vi "Test.vi"() -> ()   [LabVIEW 2017]
doc: "This example shows how to create, run a script and query the script output data."
uses:
  <instrlib>/Keithley 2600 Series/Keithley 2600 Series.lvlib
panel:
  out "Graph 2":cluster{"Y":dbl[], "Y":dbl[]}[](graph)
  out "Current":string
  in  "Numeric":i32=6000
  out "Voltage":string
  out "Time":string
  in  "Source Code":string="smua.reset()\nsmua.source.limitv = 1\nSweepILinMeasureV(smua, 0.01, 0.1, 0.2, 10)\nprintbuffer(1, 10, smua.nvbuffer1)\nprint(smua.nvbuffer1.readings[10])\n"
  in  "Script Variable (myScript)":string="myScript"
  in  "VISA resource name":refnum<visa-resource-name>
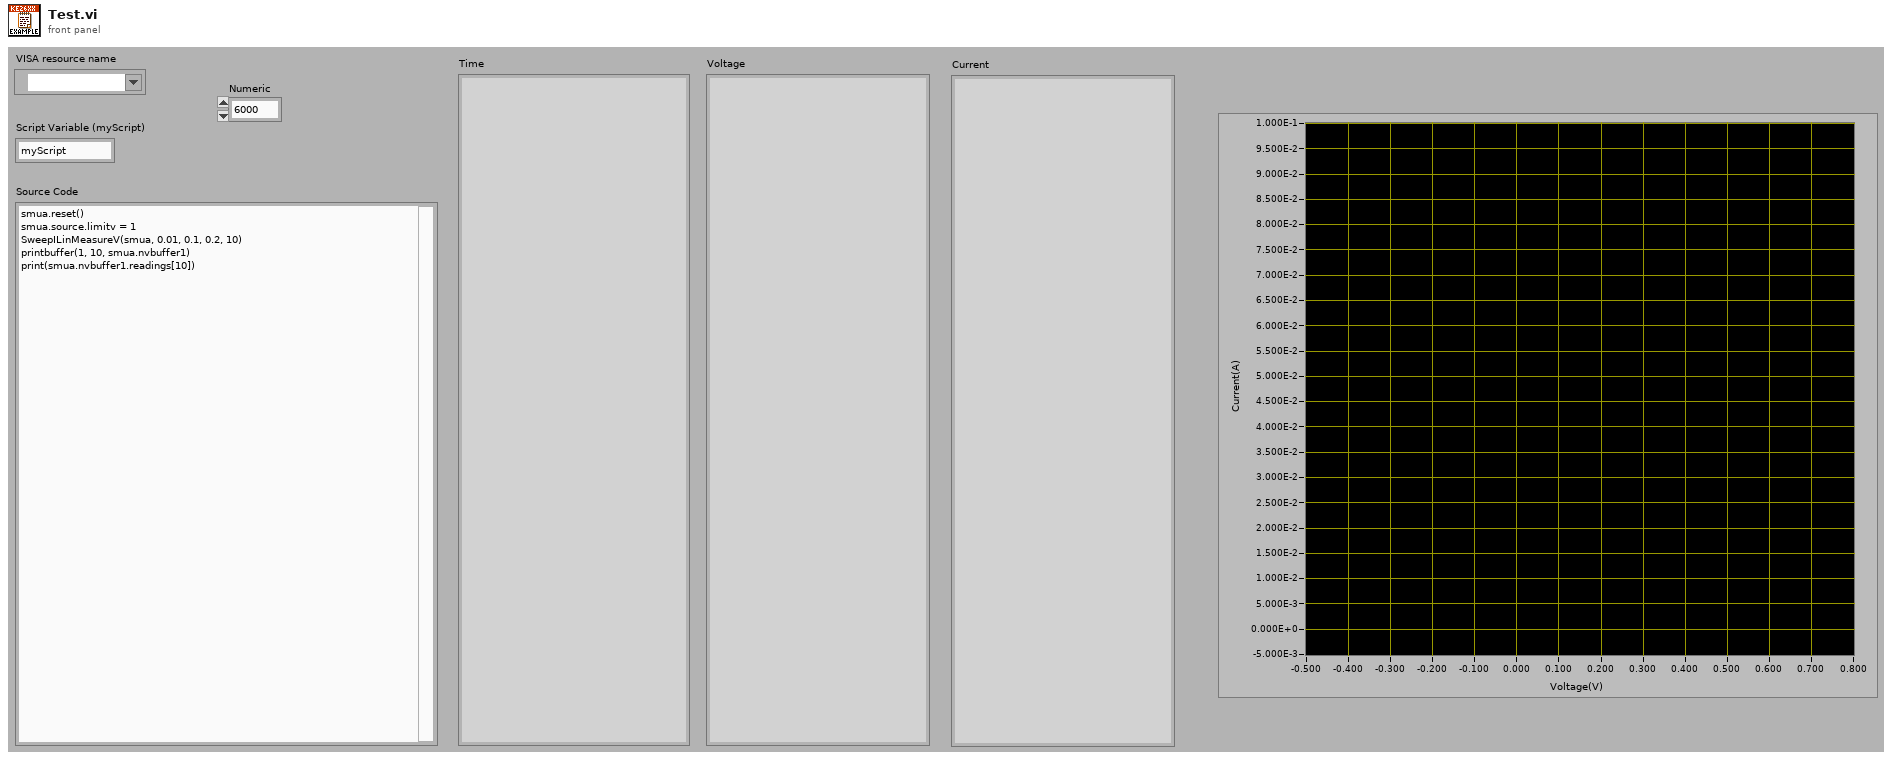
[diagram p1: front panel]
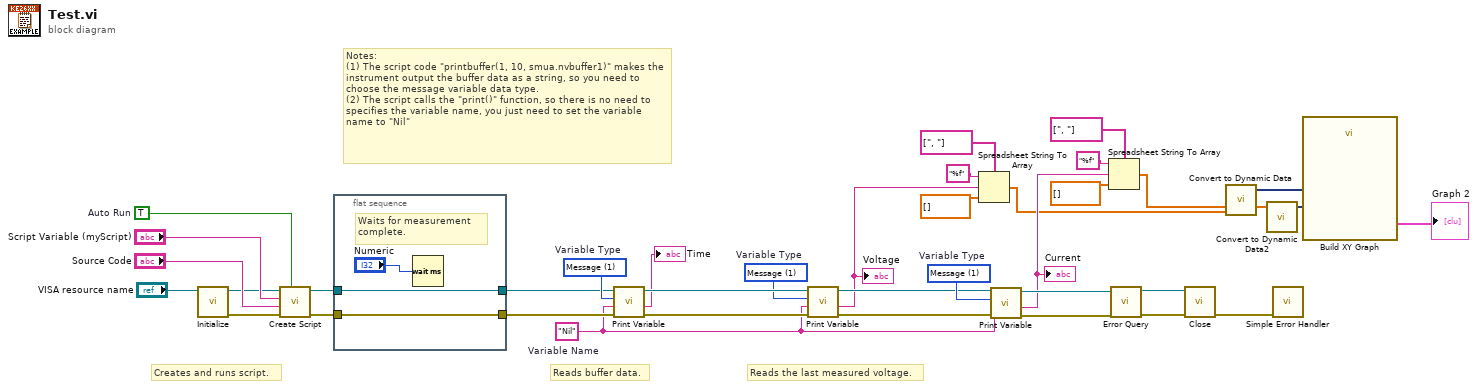
[diagram p0: block diagram]
diagram:
  w19 = 1 items=["Number", "Message"]  # Variable Type
  w30 = 1 items=["Number", "Message"]  # Variable Type
  w33 = 1 items=["Number", "Message"]  # Variable Type
  w14 = "Nil"  # Variable Name
  w34 = TRUE  # Auto Run
  # "Reads buffer data."
  # "Reads the last measured voltage."
  # "Notes: \n(1) The script code \"printbuffer(1, 10, smua.nvbuffer1)\" makes the instrument output the buffer data as a string, so you need to choose the message variable data type.\n(2) The script calls the \"print()\" function, so there is no need to specifies the variable name, you just need to set the variable name to \"Nil\""
  # "Creates and runs script."
  n1 = call <instrlib>:"Initialize.vi"("VISA resource name"="VISA resource name") -> ("error out"=w20:errorcluster, "VISA resource name out"=w21:refnum<visa-resource-name>)  [unwired: 9 in]
  n2 = call <instrlib>:"Create Script.vi"("Auto Run (F: Disable)"=w34, "error in (no error)"=w20, "Source Code"="Source Code", "Script Variable"="Script Variable (myScript)", "VISA resource name"=w21) -> ("error out"=w28:errorcluster, "VISA resource name out"=w29:refnum<visa-resource-name>)  [unwired: 5 in]
  n3 = flat-sequence {
    tunnel: w29 -> [w38]
    tunnel: w28 -> [w39]
    tunnel: [w39] -> w26
    tunnel: [w38] -> w27
    frame #0 {
      # "Waits for measurement complete."
      n4 = Wait (ms)(milliseconds to wait="Numeric") -> ()  [unwired: 1 out]
    }
  }
  n5 = call <instrlib>:"Print Variable.vi"("error in (no error)"=w26, "Variable Name"=w14, "Variable Type (0: Number)"=w33, "VISA resource name"=w27) -> ("error out"=w31:errorcluster, "Message"=→"Time":string, "VISA resource name out"=w32:refnum<visa-resource-name>)  [unwired: 4 in, 1 out]
  n6 = call <instrlib>:"Print Variable.vi"("error in (no error)"=w31, "Variable Name"=w14, "Variable Type (0: Number)"=w30, "VISA resource name"=w32) -> ("error out"=w16:errorcluster, "Message"=w11:string, "VISA resource name out"=w18:refnum<visa-resource-name>)  [unwired: 4 in, 1 out]
  "Voltage" <- w11
  n7 = Spreadsheet String To Array(delimiter (Tab)=string[] [", "], format string="%f", spreadsheet string=w11, array type (2D Dbl)=dbl[] []) -> (array=w6:dbl[])
  n8 = call <instrlib>:"Print Variable.vi"("error in (no error)"=w16, "Variable Name"=w14, "Variable Type (0: Number)"=w19, "VISA resource name"=w18) -> ("error out"=w15:errorcluster, "Message"=w8:string, "VISA resource name out"=w17:refnum<visa-resource-name>)  [unwired: 4 in, 1 out]
  "Current" <- w8
  n9 = Spreadsheet String To Array(delimiter (Tab)=string[] [", "], format string="%f", spreadsheet string=w8, array type (2D Dbl)=dbl[] []) -> (array=w4:dbl[])
  n10 = call <instrlib>:"Error Query.vi"("error in (no error)"=w15, "VISA resource name"=w17) -> ("error out"=w23:errorcluster, "VISA resource name out"=w24:refnum<visa-resource-name>)  [unwired: 6 in, 2 out]
  n11 = call <instrlib>:"Close.vi"("error in (no error)"=w23, "VISA resource name"=w24) -> ("error out"=w35:errorcluster)  [unwired: 9 in]
  n12 = call "Convert to Dynamic Data"("Array"=w6) -> ("Dynamic Data Type"=w5:dynamicdata)  [unwired: 3 in]
  n13 = call "Convert to Dynamic Data2"("Array"=w4) -> ("Dynamic Data Type"=w3:dynamicdata)  [unwired: 3 in]
  n14 = call <vilib>:"Simple Error Handler.vi"("error in (no error)"=w35) -> ()  [unwired: 4 in, 5 out]
  n15 = call "Build XY Graph"("Y Input"=w3, "X Input"=w5) -> ("XY Graph"=→"Graph 2":cluster{"X":dbl[], "Y":dbl[]}[])  [unwired: 8 in, 1 out]
